vi "letrasservo.vi"() -> ()   [LabVIEW 2016]
uses:
  <vilib>/LabVIEW Interface for Arduino/Type Defs/Board Type.ctl
  <vilib>/LabVIEW Interface for Arduino/Type Defs/Arduino Resource.ctl
  <vilib>/LabVIEW Interface for Arduino/LabVIEW Interface for Arduino.lvlib
panel:
  in  "Cluster":cluster{"String":string, "OK Button":bool}
  in  "Stop Button":bool
  out "error out":errorcluster
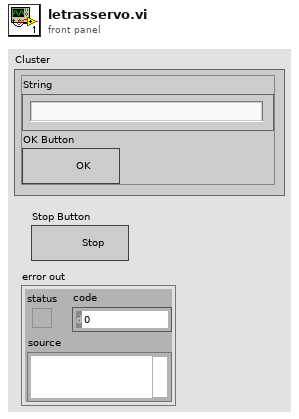
[diagram p1: front panel]
types:
  T1 = typedef "LabVIEW Interface for Arduino.lvlib/Board Type.ctl" = enum16{"Uno", "Dimuelanove w/Atmega 328", "Mega 2560"}
  T2 = typedef "LabVIEW Interface for Arduino.lvlib/Arduino Resource.ctl" = cluster{"VISA resource":refnum<visa-resource-name>, "Board Type":T1, "Connection Type":enum8{"USB / Serial"}, "Bytes Per Packet (15)":u8}
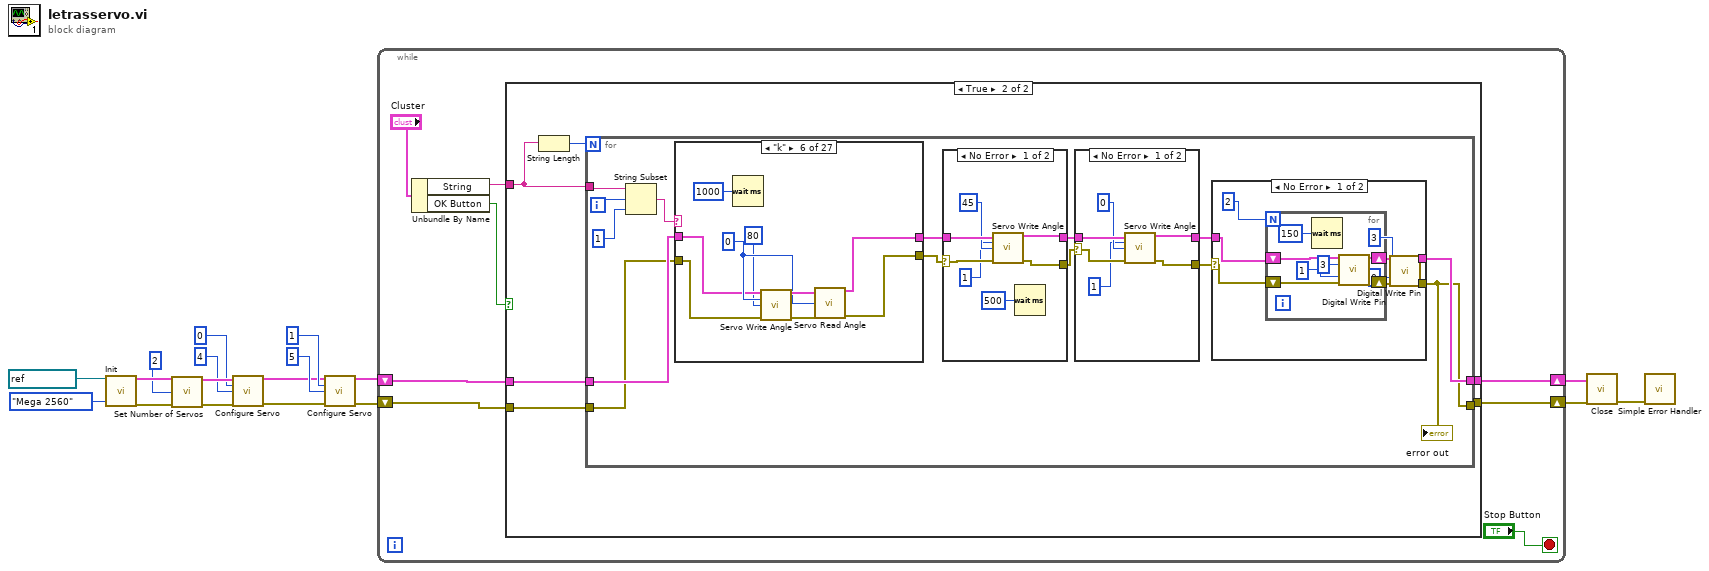
[diagram p0: block diagram]
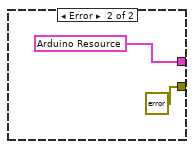
[diagram p5: hidden frame]
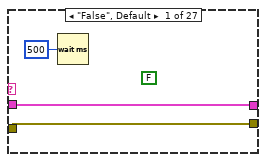
[diagram p6: hidden frame]
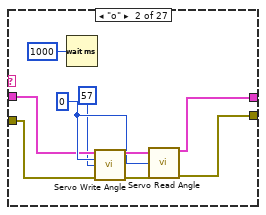
[diagram p7: hidden frame]
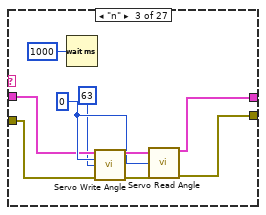
[diagram p8: hidden frame]
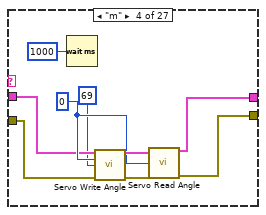
[diagram p9: hidden frame]
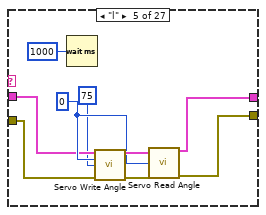
[diagram p10: hidden frame]
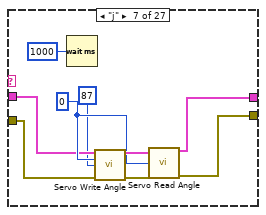
[diagram p11: hidden frame]
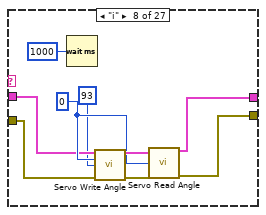
[diagram p12: hidden frame]
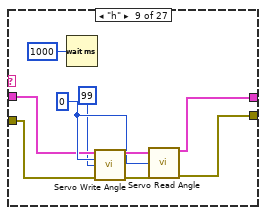
[diagram p13: hidden frame]
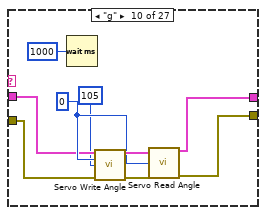
[diagram p14: hidden frame]
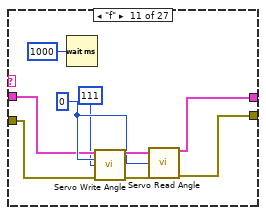
[diagram p15: hidden frame]
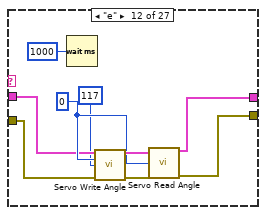
[diagram p16: hidden frame]
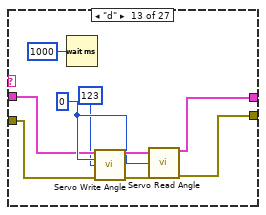
[diagram p17: hidden frame]
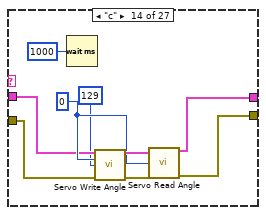
[diagram p18: hidden frame]
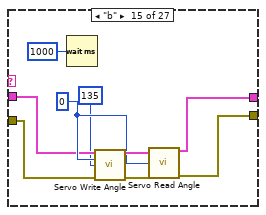
[diagram p19: hidden frame]
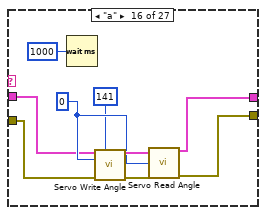
[diagram p20: hidden frame]
diagram:
  n1 = call <vilib>:"Init.vi"("VISA resource"=refnum<visa-resource-name> "COM16", "Board Type (Uno)"=Board_Type."Mega 2560") -> ("Arduino Resource"=w18:T2, "error out"=w17:errorcluster)  [unwired: 16 in]
  n2 = call <vilib>:"Set Number of Servos.vi"("Arduino Resource"=w18, "Number Of Servos (1)"=u8 2 ("Number of Servos"), "error in"=w17) -> ("Arduino Resource"=w15:T2, "error out"=w14:errorcluster)  [unwired: 11 in]
  n3 = call <vilib>:"Configure Servo.vi"("Arduino Resource"=w15, "Servo Number (0)"=u8 0 ("Servo Number"), "DIO Pin (2)"=u8 4 ("Servo Number"), "error in"=w14) -> ("Arduino Resource"=w4:T2, "error out"=w3:errorcluster)  [unwired: 10 in]
  n4 = call <vilib>:"Configure Servo.vi"("Arduino Resource"=w4, "Servo Number (0)"=u8 1 ("Servo Number"), "DIO Pin (2)"=u8 5 ("Servo Number"), "error in"=w3) -> ("Arduino Resource"=w2:T2, "error out"=w1:errorcluster)  [unwired: 10 in]
  n5 = while {
    shift-right: [w23] -> w7
    shift-left: w2 -> [w26]
    shift-right: [w24] -> w8
    shift-left: w1 -> [w25]
    stop <- "Stop Button" stop-if-true
    n6 = Unbundle By Name("Cluster") -> ("String"=w21:string, "OK Button"=w20:bool)
    n7 = case shown="True" w20 {
      tunnel: w21 -> [_ w34]
      tunnel: w26 -> [w28 w33]
      tunnel: w25 -> [w27 w32]
      tunnel: [w27 w31] -> w24
      tunnel: [w28 w30] -> w23
      frame False {
      }
      frame True {
        n8 = String Length(string=w34) -> (length=w29:i32)
        n9 = for {
          N: w29 -> [_]
          tunnel: w34 -> [w48]
          tunnel: w33 -> [w42]
          tunnel: w32 -> [w41]
          tunnel: [w43] -> w31
          tunnel: [w44] -> w30
          i -> [w46]
          n10 = String Subset(string=w48, offset (0)=w46, length (rest)=1 ("length (rest)")) -> (substring=w45:string)
          n11 = case shown="\"k\"" w45 {
            tunnel: w42 -> [w85 w91 w100 w109 w118 w127 w136 w145 w154 w163 w172 w181 w190 w199 w208 w217 w226 w235 w244 w253 w262 w271 w280 w289 w298 w307 w316]
            tunnel: w41 -> [w84 w90 w99 w108 w117 w126 w135 w144 w153 w162 w171 w180 w189 w198 w207 w216 w225 w234 w243 w252 w261 w270 w279 w288 w297 w306 w315]
            tunnel: [w85 w89 w98 w107 w116 w125 w134 w143 w152 w161 w170 w179 w188 w197 w206 w215 w224 w233 w242 w251 w260 w269 w278 w287 w296 w305 w314] -> w40
            tunnel: [w84 w88 w97 w106 w115 w124 w133 w142 w151 w160 w169 w178 w187 w196 w205 w214 w223 w232 w241 w250 w259 w268 w277 w286 w295 w304 w313] -> w39
            frame "False", Default {
              (unwired) FALSE
              n12 = Wait (ms)(milliseconds to wait=u32 500) -> ()  [unwired: 1 out]
            }
            frame "o" {
              w92 = u8 0 ("Servo Number")
              n13 = Wait (ms)(milliseconds to wait=u32 1000) -> ()  [unwired: 1 out]
              n14 = call <vilib>:"Servo Write Angle.vi"("Arduino Resource"=w91, "Servo Number"=w92, "Angle (Degrees)"=57, "error in"=w90) -> ("Arduino Resource"=w94:T2, "error out"=w93:errorcluster)  [unwired: 10 in]
              n15 = call <vilib>:"Servo Read Angle.vi"("Arduino Resource"=w94, "Servo Number"=w92, "error in"=w93) -> ("Arduino Resource"=w89:T2, "error out"=w88:errorcluster)  [unwired: 10 in, 1 out]
            }
            frame "n" {
              w101 = u8 0 ("Servo Number")
              n16 = Wait (ms)(milliseconds to wait=u32 1000) -> ()  [unwired: 1 out]
              n17 = call <vilib>:"Servo Write Angle.vi"("Arduino Resource"=w100, "Servo Number"=w101, "Angle (Degrees)"=63, "error in"=w99) -> ("Arduino Resource"=w103:T2, "error out"=w102:errorcluster)  [unwired: 10 in]
              n18 = call <vilib>:"Servo Read Angle.vi"("Arduino Resource"=w103, "Servo Number"=w101, "error in"=w102) -> ("Arduino Resource"=w98:T2, "error out"=w97:errorcluster)  [unwired: 10 in, 1 out]
            }
            frame "m" {
              w110 = u8 0 ("Servo Number")
              n19 = Wait (ms)(milliseconds to wait=u32 1000) -> ()  [unwired: 1 out]
              n20 = call <vilib>:"Servo Write Angle.vi"("Arduino Resource"=w109, "Servo Number"=w110, "Angle (Degrees)"=69, "error in"=w108) -> ("Arduino Resource"=w112:T2, "error out"=w111:errorcluster)  [unwired: 10 in]
              n21 = call <vilib>:"Servo Read Angle.vi"("Arduino Resource"=w112, "Servo Number"=w110, "error in"=w111) -> ("Arduino Resource"=w107:T2, "error out"=w106:errorcluster)  [unwired: 10 in, 1 out]
            }
            frame "l" {
              w119 = u8 0 ("Servo Number")
              n22 = Wait (ms)(milliseconds to wait=u32 1000) -> ()  [unwired: 1 out]
              n23 = call <vilib>:"Servo Write Angle.vi"("Arduino Resource"=w118, "Servo Number"=w119, "Angle (Degrees)"=75, "error in"=w117) -> ("Arduino Resource"=w121:T2, "error out"=w120:errorcluster)  [unwired: 10 in]
              n24 = call <vilib>:"Servo Read Angle.vi"("Arduino Resource"=w121, "Servo Number"=w119, "error in"=w120) -> ("Arduino Resource"=w116:T2, "error out"=w115:errorcluster)  [unwired: 10 in, 1 out]
            }
            frame "k" {
              w128 = u8 0 ("Servo Number")
              n25 = Wait (ms)(milliseconds to wait=u32 1000) -> ()  [unwired: 1 out]
              n26 = call <vilib>:"Servo Write Angle.vi"("Arduino Resource"=w127, "Servo Number"=w128, "Angle (Degrees)"=80, "error in"=w126) -> ("Arduino Resource"=w130:T2, "error out"=w129:errorcluster)  [unwired: 10 in]
              n27 = call <vilib>:"Servo Read Angle.vi"("Arduino Resource"=w130, "Servo Number"=w128, "error in"=w129) -> ("Arduino Resource"=w125:T2, "error out"=w124:errorcluster)  [unwired: 10 in, 1 out]
            }
            frame "j" {
              w137 = u8 0 ("Servo Number")
              n28 = Wait (ms)(milliseconds to wait=u32 1000) -> ()  [unwired: 1 out]
              n29 = call <vilib>:"Servo Write Angle.vi"("Arduino Resource"=w136, "Servo Number"=w137, "Angle (Degrees)"=87, "error in"=w135) -> ("Arduino Resource"=w139:T2, "error out"=w138:errorcluster)  [unwired: 10 in]
              n30 = call <vilib>:"Servo Read Angle.vi"("Arduino Resource"=w139, "Servo Number"=w137, "error in"=w138) -> ("Arduino Resource"=w134:T2, "error out"=w133:errorcluster)  [unwired: 10 in, 1 out]
            }
            frame "i" {
              w146 = u8 0 ("Servo Number")
              n31 = Wait (ms)(milliseconds to wait=u32 1000) -> ()  [unwired: 1 out]
              n32 = call <vilib>:"Servo Write Angle.vi"("Arduino Resource"=w145, "Servo Number"=w146, "Angle (Degrees)"=93, "error in"=w144) -> ("Arduino Resource"=w148:T2, "error out"=w147:errorcluster)  [unwired: 10 in]
              n33 = call <vilib>:"Servo Read Angle.vi"("Arduino Resource"=w148, "Servo Number"=w146, "error in"=w147) -> ("Arduino Resource"=w143:T2, "error out"=w142:errorcluster)  [unwired: 10 in, 1 out]
            }
            frame "h" {
              w155 = u8 0 ("Servo Number")
              n34 = Wait (ms)(milliseconds to wait=u32 1000) -> ()  [unwired: 1 out]
              n35 = call <vilib>:"Servo Write Angle.vi"("Arduino Resource"=w154, "Servo Number"=w155, "Angle (Degrees)"=99, "error in"=w153) -> ("Arduino Resource"=w157:T2, "error out"=w156:errorcluster)  [unwired: 10 in]
              n36 = call <vilib>:"Servo Read Angle.vi"("Arduino Resource"=w157, "Servo Number"=w155, "error in"=w156) -> ("Arduino Resource"=w152:T2, "error out"=w151:errorcluster)  [unwired: 10 in, 1 out]
            }
            frame "g" {
              w164 = u8 0 ("Servo Number")
              n37 = Wait (ms)(milliseconds to wait=u32 1000) -> ()  [unwired: 1 out]
              n38 = call <vilib>:"Servo Write Angle.vi"("Arduino Resource"=w163, "Servo Number"=w164, "Angle (Degrees)"=105, "error in"=w162) -> ("Arduino Resource"=w166:T2, "error out"=w165:errorcluster)  [unwired: 10 in]
              n39 = call <vilib>:"Servo Read Angle.vi"("Arduino Resource"=w166, "Servo Number"=w164, "error in"=w165) -> ("Arduino Resource"=w161:T2, "error out"=w160:errorcluster)  [unwired: 10 in, 1 out]
            }
            frame "f" {
              w173 = u8 0 ("Servo Number")
              n40 = Wait (ms)(milliseconds to wait=u32 1000) -> ()  [unwired: 1 out]
              n41 = call <vilib>:"Servo Write Angle.vi"("Arduino Resource"=w172, "Servo Number"=w173, "Angle (Degrees)"=111, "error in"=w171) -> ("Arduino Resource"=w175:T2, "error out"=w174:errorcluster)  [unwired: 10 in]
              n42 = call <vilib>:"Servo Read Angle.vi"("Arduino Resource"=w175, "Servo Number"=w173, "error in"=w174) -> ("Arduino Resource"=w170:T2, "error out"=w169:errorcluster)  [unwired: 10 in, 1 out]
            }
            frame "e" {
              w182 = u8 0 ("Servo Number")
              n43 = Wait (ms)(milliseconds to wait=u32 1000) -> ()  [unwired: 1 out]
              n44 = call <vilib>:"Servo Write Angle.vi"("Arduino Resource"=w181, "Servo Number"=w182, "Angle (Degrees)"=117, "error in"=w180) -> ("Arduino Resource"=w184:T2, "error out"=w183:errorcluster)  [unwired: 10 in]
              n45 = call <vilib>:"Servo Read Angle.vi"("Arduino Resource"=w184, "Servo Number"=w182, "error in"=w183) -> ("Arduino Resource"=w179:T2, "error out"=w178:errorcluster)  [unwired: 10 in, 1 out]
            }
            frame "d" {
              w191 = u8 0 ("Servo Number")
              n46 = Wait (ms)(milliseconds to wait=u32 1000) -> ()  [unwired: 1 out]
              n47 = call <vilib>:"Servo Write Angle.vi"("Arduino Resource"=w190, "Servo Number"=w191, "Angle (Degrees)"=123, "error in"=w189) -> ("Arduino Resource"=w193:T2, "error out"=w192:errorcluster)  [unwired: 10 in]
              n48 = call <vilib>:"Servo Read Angle.vi"("Arduino Resource"=w193, "Servo Number"=w191, "error in"=w192) -> ("Arduino Resource"=w188:T2, "error out"=w187:errorcluster)  [unwired: 10 in, 1 out]
            }
            frame "c" {
              w200 = u8 0 ("Servo Number")
              n49 = Wait (ms)(milliseconds to wait=u32 1000) -> ()  [unwired: 1 out]
              n50 = call <vilib>:"Servo Write Angle.vi"("Arduino Resource"=w199, "Servo Number"=w200, "Angle (Degrees)"=129, "error in"=w198) -> ("Arduino Resource"=w202:T2, "error out"=w201:errorcluster)  [unwired: 10 in]
              n51 = call <vilib>:"Servo Read Angle.vi"("Arduino Resource"=w202, "Servo Number"=w200, "error in"=w201) -> ("Arduino Resource"=w197:T2, "error out"=w196:errorcluster)  [unwired: 10 in, 1 out]
            }
            frame "b" {
              w209 = u8 0 ("Servo Number")
              n52 = Wait (ms)(milliseconds to wait=u32 1000) -> ()  [unwired: 1 out]
              n53 = call <vilib>:"Servo Write Angle.vi"("Arduino Resource"=w208, "Servo Number"=w209, "Angle (Degrees)"=135, "error in"=w207) -> ("Arduino Resource"=w211:T2, "error out"=w210:errorcluster)  [unwired: 10 in]
              n54 = call <vilib>:"Servo Read Angle.vi"("Arduino Resource"=w211, "Servo Number"=w209, "error in"=w210) -> ("Arduino Resource"=w206:T2, "error out"=w205:errorcluster)  [unwired: 10 in, 1 out]
            }
            frame "a" {
              w218 = u8 0 ("Servo Number")
              n55 = Wait (ms)(milliseconds to wait=u32 1000) -> ()  [unwired: 1 out]
              n56 = call <vilib>:"Servo Write Angle.vi"("Arduino Resource"=w217, "Servo Number"=w218, "Angle (Degrees)"=141, "error in"=w216) -> ("Arduino Resource"=w220:T2, "error out"=w219:errorcluster)  [unwired: 10 in]
              n57 = call <vilib>:"Servo Read Angle.vi"("Arduino Resource"=w220, "Servo Number"=w218, "error in"=w219) -> ("Arduino Resource"=w215:T2, "error out"=w214:errorcluster)  [unwired: 10 in, 1 out]
            }
            frame "s" {
              w227 = u8 0 ("Servo Number")
              n58 = Wait (ms)(milliseconds to wait=u32 1000) -> ()  [unwired: 1 out]
              n59 = call <vilib>:"Servo Write Angle.vi"("Arduino Resource"=w226, "Servo Number"=w227, "Angle (Degrees)"=43, "error in"=w225) -> ("Arduino Resource"=w229:T2, "error out"=w228:errorcluster)  [unwired: 10 in]
              n60 = call <vilib>:"Servo Read Angle.vi"("Arduino Resource"=w229, "Servo Number"=w227, "error in"=w228) -> ("Arduino Resource"=w224:T2, "error out"=w223:errorcluster)  [unwired: 10 in, 1 out]
            }
            frame "z" {
              w236 = u8 0 ("Servo Number")
              n61 = Wait (ms)(milliseconds to wait=u32 1000) -> ()  [unwired: 1 out]
              n62 = call <vilib>:"Servo Write Angle.vi"("Arduino Resource"=w235, "Servo Number"=w236, "Angle (Degrees)"=1, "error in"=w234) -> ("Arduino Resource"=w238:T2, "error out"=w237:errorcluster)  [unwired: 10 in]
              n63 = call <vilib>:"Servo Read Angle.vi"("Arduino Resource"=w238, "Servo Number"=w236, "error in"=w237) -> ("Arduino Resource"=w233:T2, "error out"=w232:errorcluster)  [unwired: 10 in, 1 out]
            }
            frame "y" {
              w245 = u8 0 ("Servo Number")
              n64 = Wait (ms)(milliseconds to wait=u32 1000) -> ()  [unwired: 1 out]
              n65 = call <vilib>:"Servo Write Angle.vi"("Arduino Resource"=w244, "Servo Number"=w245, "Angle (Degrees)"=3, "error in"=w243) -> ("Arduino Resource"=w247:T2, "error out"=w246:errorcluster)  [unwired: 10 in]
              n66 = call <vilib>:"Servo Read Angle.vi"("Arduino Resource"=w247, "Servo Number"=w245, "error in"=w246) -> ("Arduino Resource"=w242:T2, "error out"=w241:errorcluster)  [unwired: 10 in, 1 out]
            }
            frame "x" {
              w254 = u8 0 ("Servo Number")
              n67 = Wait (ms)(milliseconds to wait=u32 1000) -> ()  [unwired: 1 out]
              n68 = call <vilib>:"Servo Write Angle.vi"("Arduino Resource"=w253, "Servo Number"=w254, "Angle (Degrees)"=9, "error in"=w252) -> ("Arduino Resource"=w256:T2, "error out"=w255:errorcluster)  [unwired: 10 in]
              n69 = call <vilib>:"Servo Read Angle.vi"("Arduino Resource"=w256, "Servo Number"=w254, "error in"=w255) -> ("Arduino Resource"=w251:T2, "error out"=w250:errorcluster)  [unwired: 10 in, 1 out]
            }
            frame "w" {
              w263 = u8 0 ("Servo Number")
              n70 = Wait (ms)(milliseconds to wait=u32 1000) -> ()  [unwired: 1 out]
              n71 = call <vilib>:"Servo Write Angle.vi"("Arduino Resource"=w262, "Servo Number"=w263, "Angle (Degrees)"=15, "error in"=w261) -> ("Arduino Resource"=w265:T2, "error out"=w264:errorcluster)  [unwired: 10 in]
              n72 = call <vilib>:"Servo Read Angle.vi"("Arduino Resource"=w265, "Servo Number"=w263, "error in"=w264) -> ("Arduino Resource"=w260:T2, "error out"=w259:errorcluster)  [unwired: 10 in, 1 out]
            }
            frame "v" {
              w272 = u8 0 ("Servo Number")
              n73 = Wait (ms)(milliseconds to wait=u32 1000) -> ()  [unwired: 1 out]
              n74 = call <vilib>:"Servo Write Angle.vi"("Arduino Resource"=w271, "Servo Number"=w272, "Angle (Degrees)"=21, "error in"=w270) -> ("Arduino Resource"=w274:T2, "error out"=w273:errorcluster)  [unwired: 10 in]
              n75 = call <vilib>:"Servo Read Angle.vi"("Arduino Resource"=w274, "Servo Number"=w272, "error in"=w273) -> ("Arduino Resource"=w269:T2, "error out"=w268:errorcluster)  [unwired: 10 in, 1 out]
            }
            frame "u" {
              w281 = u8 0 ("Servo Number")
              n76 = Wait (ms)(milliseconds to wait=u32 1000) -> ()  [unwired: 1 out]
              n77 = call <vilib>:"Servo Write Angle.vi"("Arduino Resource"=w280, "Servo Number"=w281, "Angle (Degrees)"=27, "error in"=w279) -> ("Arduino Resource"=w283:T2, "error out"=w282:errorcluster)  [unwired: 10 in]
              n78 = call <vilib>:"Servo Read Angle.vi"("Arduino Resource"=w283, "Servo Number"=w281, "error in"=w282) -> ("Arduino Resource"=w278:T2, "error out"=w277:errorcluster)  [unwired: 10 in, 1 out]
            }
            frame "t" {
              w290 = u8 0 ("Servo Number")
              n79 = Wait (ms)(milliseconds to wait=u32 1000) -> ()  [unwired: 1 out]
              n80 = call <vilib>:"Servo Write Angle.vi"("Arduino Resource"=w289, "Servo Number"=w290, "Angle (Degrees)"=33, "error in"=w288) -> ("Arduino Resource"=w292:T2, "error out"=w291:errorcluster)  [unwired: 10 in]
              n81 = call <vilib>:"Servo Read Angle.vi"("Arduino Resource"=w292, "Servo Number"=w290, "error in"=w291) -> ("Arduino Resource"=w287:T2, "error out"=w286:errorcluster)  [unwired: 10 in, 1 out]
            }
            frame "r" {
              w299 = u8 0 ("Servo Number")
              n82 = Wait (ms)(milliseconds to wait=u32 1000) -> ()  [unwired: 1 out]
              n83 = call <vilib>:"Servo Write Angle.vi"("Arduino Resource"=w298, "Servo Number"=w299, "Angle (Degrees)"=39, "error in"=w297) -> ("Arduino Resource"=w301:T2, "error out"=w300:errorcluster)  [unwired: 10 in]
              n84 = call <vilib>:"Servo Read Angle.vi"("Arduino Resource"=w301, "Servo Number"=w299, "error in"=w300) -> ("Arduino Resource"=w296:T2, "error out"=w295:errorcluster)  [unwired: 10 in, 1 out]
            }
            frame "q" {
              w308 = u8 0 ("Servo Number")
              n85 = Wait (ms)(milliseconds to wait=u32 1000) -> ()  [unwired: 1 out]
              n86 = call <vilib>:"Servo Write Angle.vi"("Arduino Resource"=w307, "Servo Number"=w308, "Angle (Degrees)"=45, "error in"=w306) -> ("Arduino Resource"=w310:T2, "error out"=w309:errorcluster)  [unwired: 10 in]
              n87 = call <vilib>:"Servo Read Angle.vi"("Arduino Resource"=w310, "Servo Number"=w308, "error in"=w309) -> ("Arduino Resource"=w305:T2, "error out"=w304:errorcluster)  [unwired: 10 in, 1 out]
            }
            frame "p" {
              w317 = u8 0 ("Servo Number")
              n88 = Wait (ms)(milliseconds to wait=u32 1000) -> ()  [unwired: 1 out]
              n89 = call <vilib>:"Servo Write Angle.vi"("Arduino Resource"=w316, "Servo Number"=w317, "Angle (Degrees)"=51, "error in"=w315) -> ("Arduino Resource"=w319:T2, "error out"=w318:errorcluster)  [unwired: 10 in]
              n90 = call <vilib>:"Servo Read Angle.vi"("Arduino Resource"=w319, "Servo Number"=w317, "error in"=w318) -> ("Arduino Resource"=w314:T2, "error out"=w313:errorcluster)  [unwired: 10 in, 1 out]
            }
          }
          n91 = case shown="No Error" w39 {
            selector: w39 -> [w61 w64]
            tunnel: [w62 w65] -> w38
            tunnel: w40 -> [w63 w65]
            tunnel: [w60 w64] -> w37
            frame No Error {
              n92 = call <vilib>:"Servo Write Angle.vi"("Arduino Resource"=w63, "Servo Number"=u8 1, "Angle (Degrees)"=u8 45, "error in"=w61) -> ("Arduino Resource"=w62:T2, "error out"=w60:errorcluster)  [unwired: 10 in]
              n93 = Wait (ms)(milliseconds to wait=u32 500) -> ()  [unwired: 1 out]
            }
            frame Error {
            }
          }
          n94 = case shown="No Error" w37 {
            selector: w37 -> [w52 w55]
            tunnel: [w53 w56] -> w36
            tunnel: w38 -> [w54 w56]
            tunnel: [w51 w55] -> w35
            frame No Error {
              n95 = call <vilib>:"Servo Write Angle.vi"("Arduino Resource"=w54, "Servo Number"=u8 1, "Angle (Degrees)"=u8 0, "error in"=w52) -> ("Arduino Resource"=w53:T2, "error out"=w51:errorcluster)  [unwired: 10 in]
            }
            frame Error {
            }
          }
          n96 = case shown="No Error" w35 {
            selector: w35 -> [w67 _]
            tunnel: [w73 T2 {"VISA resource"="", "Board Type"=enum."Uno", "Connection Type"=enum."USB / Serial", "Bytes Per Packet (15)"=15} ("Arduino Resource")] -> w44
            tunnel: [w72 errorcluster {"status"=FALSE, "code"=0, "source"=""} ("error out")] -> w43
            tunnel: w36 -> [w66 _]
            frame No Error {
              n97 = for {
                N: 2 -> [_]
                shift-right: [w79] -> w74
                shift-left: w66 -> [w81]
                shift-right: [w78] -> w71
                shift-left: w67 -> [w80]
                n98 = Wait (ms)(milliseconds to wait=u32 150) -> ()  [unwired: 1 out]
                n99 = call <vilib>:"Digital Write Pin.vi"("Arduino Resource"=w81, "Digital I/O Pin (0)"=u8 3, "Value (0)"=u8 1, "error in"=w80) -> ("Arduino Resource"=w79:T2, "error out"=w78:errorcluster)  [unwired: 10 in]
              }
              n100 = call <vilib>:"Digital Write Pin.vi"("Arduino Resource"=w74, "Digital I/O Pin (0)"=u8 3, "Value (0)"=u8 0, "error in"=w71) -> ("Arduino Resource"=w73:T2, "error out"=w72:errorcluster)  [unwired: 10 in]
            }
            frame Error {
            }
          }
          "error out" <- w43
        }
      }
    }
  }
  n101 = call <vilib>:"Close.vi"("Arduino Resource"=w7, "error in"=w8) -> ("error out"=w10:errorcluster)  [unwired: 13 in]
  n102 = call <vilib>:"Simple Error Handler.vi"("error in (no error)"=w10) -> ()  [unwired: 4 in, 5 out]
